vi "calculateTimeStep.vi"(8 "error in (no error)":errorcluster, 11 "RampEvent in":refnum<class "RampEvent.lvclass">) -> (0 "error out":errorcluster, 1 "valueStep":dbl, 2 "timeStep":dbl, 3 "RampEvent out":refnum<class "RampEvent.lvclass">, 4 "number of Steps":i32)   [LabVIEW 2011, in "Tools.lvlib" / "Scripting.lvlib" / "RampEvent.lvclass"]
uses:
  RampEvent.lvclass
  RampEvent.lvclass/RampEvent.ctl
  ScriptEvent.lvclass
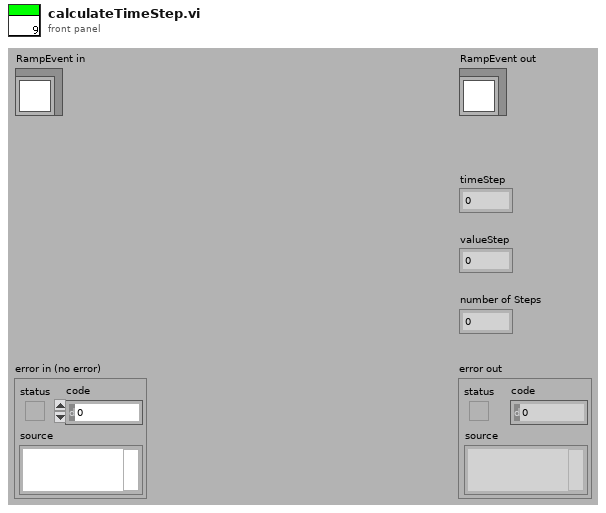
[diagram p1: front panel]
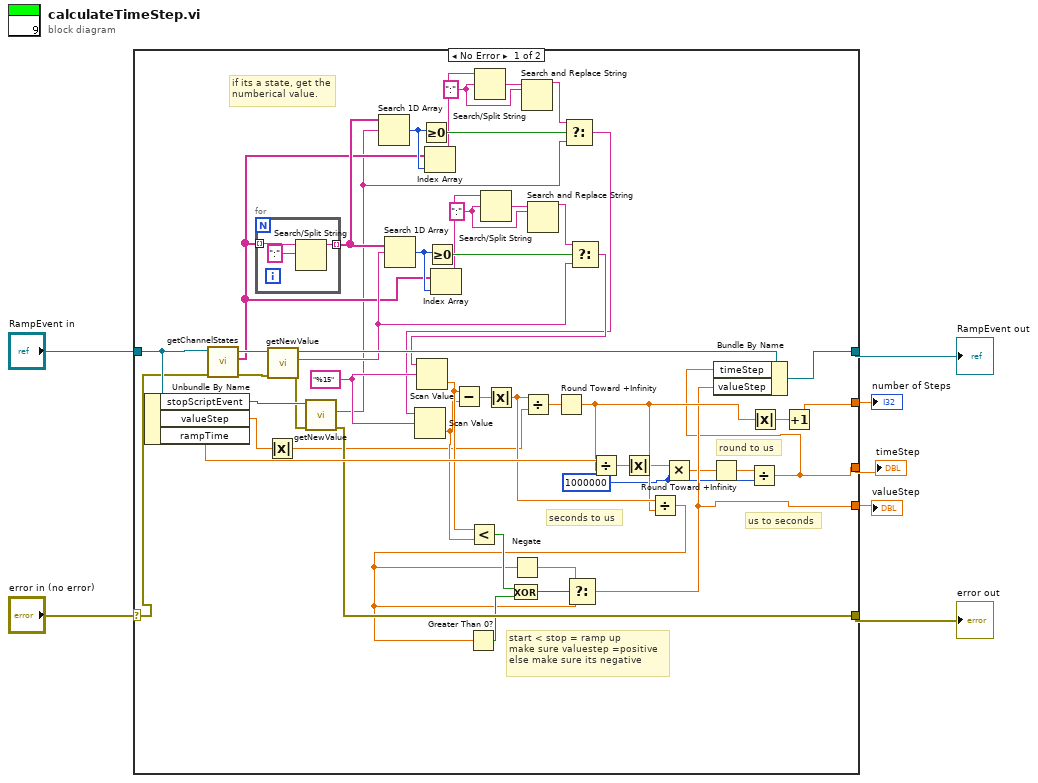
[diagram p0: block diagram]
diagram:
  n1 = case shown="No Error" "error in (no error)" {
    selector: "error in (no error)" -> [w47 w63]
    tunnel: [w50 w63] -> w6
    tunnel: [w51 w62] -> w4
    tunnel: "RampEvent in" -> [w49 w62]
    tunnel: [w8 _] -> w3
    tunnel: [w13 _] -> w2
    tunnel: [w16 _] -> w1
    frame No Error {
      w9 = 1000000
      w33 = ":"
      w41 = ":"
      w56 = "%15"
      # "round to us"
      # "us to seconds"
      # "seconds to us"
      # "start < stop = ramp up\nmake sure valuestep =positive\nelse make sure its negative"
      # "if its a state, get the\nnumberical value."
      n2 = Unbundle By Name(w49) -> ("stopScriptEvent"=w58:refnum<class "ScriptEvent.lvclass">, "valueStep"=w15:dbl, "rampTime"=w55:dbl)
      n3 = call-dynamic "getChannelStates.vi"("error in (no error)"=w47, "ScriptEvent in"=w49) -> ("error out"=w46:errorcluster, "statesValues"=w30:string[], "ScriptEvent out"=w48:refnum<class "RampEvent.lvclass">)  [unwired: 7 in]
      n4 = for {
        tunnel: w30 -> [w61] mode=indexing
        tunnel: [w59] -> w31 mode=indexing
        n5 = Search/Split String(string=w61, search string/char (-)=":") -> (substring before match=w59:string)  [unwired: 1 in, 2 out]
      }
      n6 = Absolute Value(x=w15) -> (abs(x)=w14:dbl)
      n7 = call "getNewValue.vi"("error in (no error)"=w46, "ScriptEvent.lvclass in"=w48) -> ("error out"=w57:errorcluster, "newValue"=w39:string, "ScriptEvent.lvclass out"=w52:refnum<class "RampEvent.lvclass">)  [unwired: 7 in]
      n8 = call "getNewValue.vi"("error in (no error)"=w57, "ScriptEvent.lvclass in"=w58) -> ("error out"=w50:errorcluster, "newValue"=w29:string)  [unwired: 7 in, 1 out]
      n9 = Search 1D Array(1D array=w31, element=w29) -> (index of element=w37:i32)  [unwired: 1 in]
      n10 = Search 1D Array(1D array=w31, element=w39) -> (index of element=w45:i32)  [unwired: 1 in]
      n11 = Greater Or Equal To 0?(x=w37) -> (x >= 0?=w36:bool)
      n12 = Index Array(array=w30, index=w37) -> (element=w35:string)
      n13 = Greater Or Equal To 0?(x=w45) -> (x >= 0?=w44:bool)
      n14 = Index Array(array=w30, index=w45) -> (element=w43:string)
      n15 = Search/Split String(string=w35, search string/char (-)=w33) -> (match + rest of string=w34:string)  [unwired: 1 in, 2 out]
      n16 = Search/Split String(string=w43, search string/char (-)=w41) -> (match + rest of string=w42:string)  [unwired: 1 in, 2 out]
      n17 = Search and Replace String(input string=w34, search string=w33) -> (result string=w32:string)  [unwired: 6 in, 3 out]
      n18 = Search and Replace String(input string=w42, search string=w41) -> (result string=w40:string)  [unwired: 6 in, 3 out]
      n19 = Select(t=w32, s=w36, f=w29) -> (s? t:f=w28:string)
      n20 = Scan Value(string=w28, format string=w56) -> (value=w19:dbl)  [unwired: 1 in, 1 out]
      n21 = Select(t=w40, s=w44, f=w39) -> (s? t:f=w38:string)
      n22 = Scan Value(string=w38, format string=w56) -> (value=w20:dbl)  [unwired: 1 in, 1 out]
      n23 = Subtract(x=w20, y=w19) -> (x-y=w24:dbl)
      n24 = Less?(x=w20, y=w19) -> (x < y?=w18:bool)
      n25 = Absolute Value(x=w24) -> (abs(x)=w53:dbl)
      n26 = Divide(x=w53, y=w14) -> (x/y=w54:dbl)
      n27 = Round Toward +Infinity(x=w54) -> (ceil(x): smallest int >= x=w27:dbl)
      n28 = Divide(x=w55, y=w27) -> (x/y=w25:dbl)
      n29 = Absolute Value(x=w25) -> (abs(x)=w12:dbl)
      n30 = Divide(x=w53, y=w27) -> (x/y=w17:dbl)
      n31 = Greater Than 0?(x=w17) -> (x > 0?=w23:bool)
      n32 = Exclusive Or(1:w23, 2:w18) -> (0:w22:bool)
      n33 = Negate(x=w17) -> (-x=w21:dbl)
      n34 = Select(t=w21, s=w22, f=w17) -> (s? t:f=w16:dbl)
      n35 = Multiply(x=w12, y=w9) -> (x*y=w11:dbl)
      n36 = Round Toward +Infinity(x=w11) -> (ceil(x): smallest int >= x=w10:dbl)
      n37 = Divide(x=w10, y=w9) -> (x/y=w8:dbl)
      n38 = Bundle By Name(cluster=w52, "timeStep"=w8, "valueStep"=w16) -> (w51:refnum<class "RampEvent.lvclass">)
      n39 = Absolute Value(x=w27) -> (abs(x)=w26:dbl)
      n40 = Increment(x=w26) -> (x+1=w13:dbl)
    }
    frame Error {
    }
  }
  "error out" <- w6
  "RampEvent out" <- w4
  "timeStep" <- w3
  "number of Steps" <- w2
  "valueStep" <- w1
